vi "OC_SC_Detection.vi"() -> (2 "Open Loop Channels Array":bool[](array[boolean]), 3 "Short Circuit Channels Array":bool[](array[boolean]))   [LabVIEW 2017, in "VDMS_VibAPI_8.lvlib"]
uses:
  <vilib>/addons/InsightCM/Devices/Shared/Cms/Fpga/AcquisitionFpgaTach/source/subVIs/VibAPI_8/VDMS_VibAPI_8.lvlib
  <vilib>/rvi/eio/common/nirviEmuTemplateMethod_errors.vi
  <vilib>/eio/EIOMethodNode/EIOMethodNode.xnode
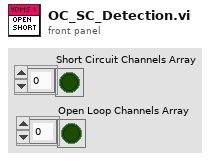
[diagram p1: front panel]
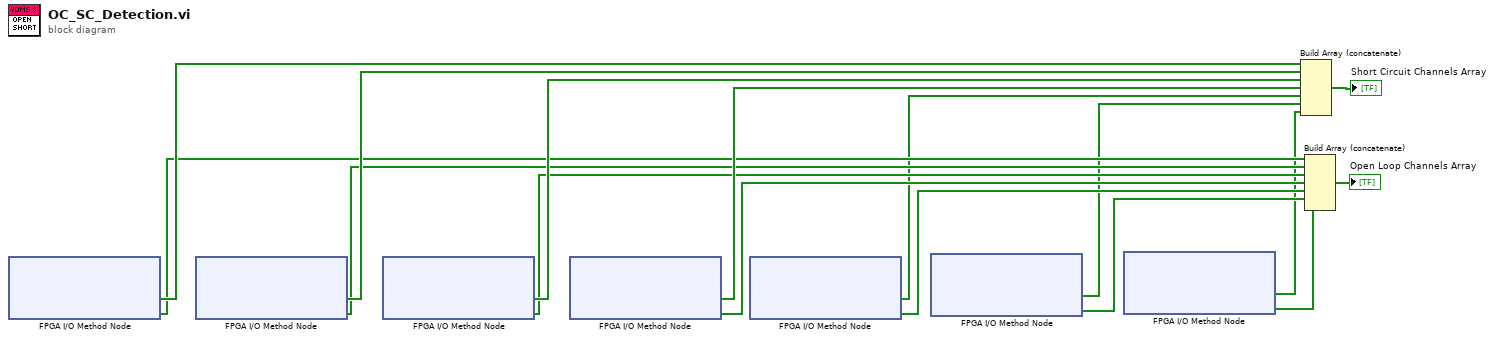
[diagram p0: block diagram]
diagram:
  n1 = xnode "FPGA I/O Method Node"() -> ("Short Circuit"=w16:bool[], "Open Loop"=w12:bool[])  [unwired: 1 in, 1 out]
  n2 = xnode "FPGA I/O Method Node"() -> ("Short Circuit"=w15:bool[], "Open Loop"=w11:bool[])  [unwired: 1 in, 1 out]
  n3 = xnode "FPGA I/O Method Node"() -> ("Short Circuit"=w14:bool[], "Open Loop"=w10:bool[])  [unwired: 1 in, 1 out]
  n4 = xnode "FPGA I/O Method Node"() -> ("Short Circuit"=w13:bool[], "Open Loop"=w9:bool[])  [unwired: 1 in, 1 out]
  n5 = xnode "FPGA I/O Method Node"() -> ("Short Circuit"=w8:bool[], "Open Loop"=w7:bool[])  [unwired: 1 in, 1 out]
  n6 = xnode "FPGA I/O Method Node"() -> ("Short Circuit"=w6:bool[], "Open Loop"=w5:bool[])  [unwired: 1 in, 1 out]
  n7 = xnode "FPGA I/O Method Node"() -> ("Short Circuit"=w4:bool[], "Open Loop"=w3:bool[])  [unwired: 1 in, 1 out]
  n8 = Build Array (concatenate)(w16, w15, w14, w13, w8, w6, w4) -> (→"Short Circuit Channels Array":bool[])
  n9 = Build Array (concatenate)(w12, w11, w10, w9, w7, w5, w3) -> (→"Open Loop Channels Array":bool[])
